vi "ep_Generate Lowpas Filter Coeficients.vi"(0 "nominal frequency":enum16{"50 Hz", "60 Hz"}(ring), 1 "restart (F)":bool, 5 "nominal sampling rate (Hz)":dbl=9600.0) -> (4 "IIR filter cluster":T1, 8 "filter delay (samples)":dbl)   [LabVIEW 2011, in "NI_EP_Power Quality.lvlib"]
uses:
  <vilib>/Analysis/3filter.llb/Filter Passband Type.ctl
  <vilib>/addons/Electrical Power/PQ/NI_EP_Power Quality.lvlib
  <vilib>/Analysis/NI_AALBase.lvlib
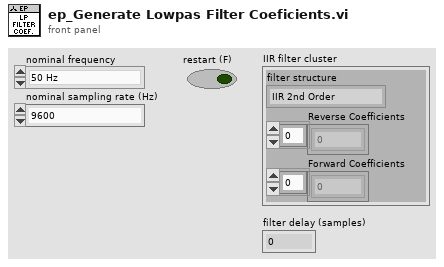
[diagram p1: front panel]
types:
  T1 = cluster{"filter structure":enum32{"IIR 2nd Order", "IIR 4th Order"}, "Reverse Coefficients":dbl[], "Forward Coefficients":dbl[]}
  T2 = typedef "NI_AALBase.lvlib/Filter Passband Type.ctl" = enum32{"Lowpass", "Highpass", "Bandpass", "Bandstop"}
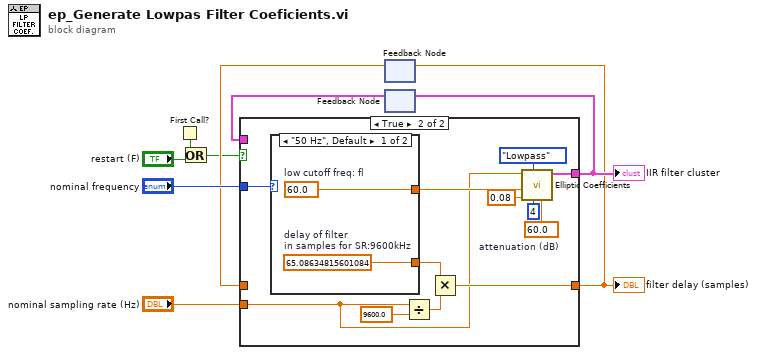
[diagram p0: block diagram]
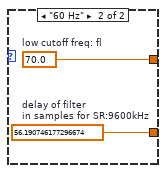
[diagram p3: hidden frame]
diagram:
  n1 = First Call?() -> (First Call?: T/F=w2:bool)
  n2 = Or(x=w2, y="restart (F)") -> (x .or. y?=w1:bool)
  n3 = feedback #1() -> (w4:dbl)  [unwired: 1 in]
  n4 = feedback #2() -> (w8:T1)  [unwired: 1 in]
  n5 = case shown="True" w1 {
    tunnel: [w11 w19] -> w9
    tunnel: w8 -> [w11 _]
    tunnel: "nominal frequency" -> [_ w15]
    tunnel: "nominal sampling rate (Hz)" -> [_ w12]
    tunnel: [w10 w13] -> w5
    tunnel: w4 -> [w10 _]
    frame False {
    }
    frame True {
      w21 = 60.0  # attenuation (dB)
      n6 = case shown="\"50 Hz\", Default" w15 {
        tunnel: [w25 w27] -> w14
        tunnel: [w24 w26] -> w18
        frame "50 Hz", Default {
          w24 = 65.08634815601084  # delay of filter in samples for SR:9600kHz
          w25 = 60.0  # low cutoff freq: fl
        }
        frame "60 Hz" {
          w26 = 56.190746177296674  # delay of filter in samples for SR:9600kHz
          w27 = 70.0  # low cutoff freq: fl
        }
      }
      n7 = Divide(x=w12, y=9600.0) -> (x/y=w17:dbl)
      n8 = Multiply(x=w18, y=w17) -> (x*y=w13:dbl)
      n9 = call <vilib>:"Elliptic Coefficients.vi"("stopband attenuation (dB)"=w21, "order"=4, "filter type"=Filter_Passband_Type."Lowpass", "passband ripple (dB)"=0.08, "low cutoff freq: fl"=w14, "sampling freq: fs"=w12) -> ("IIR Filter Cluster"=w19:T1)  [unwired: 4 in, 1 out]
    }
  }
  "IIR filter cluster" <- w9
  "filter delay (samples)" <- w5
  n10 = feedback-in #1(w5) -> ()
  n11 = feedback-in #2(w9) -> ()
